vi "labview_program_zfp_interferrometer.vi"() -> ()   [LabVIEW 2015]
uses:
  <vilib>/userdefined/High Color/IMAQdx.ctl
  <vilib>/vision/Image Controls.llb/IMAQ Image.ctl
  <vilib>/Analysis/6fits.llb/Confidence Interval (Linear).vi
  <vilib>/Utility/file.llb/Write Delimited Spreadsheet (DBL).vi
  <vilib>/Analysis/3filter.llb/Butterworth Filter (DBL).vi
  <vilib>/vision/driver/NI_Vision_Acquisition_Software.lvlib
  <resource>/objmgr/imaqdx.rc
  <vilib>/Analysis/NI_AALBase.lvlib
  <vilib>/Analysis/NI_AAL_SigProc.lvlib
  <vilib>/Analysis/NI_AALPro.lvlib
  <vilib>/ptbypt/NI_PtbyPt.lvlib
panel:
  in  "file path (use dialog)":path
  in  "prompt (Choose or enter file path)":string
  out "Intensity Graph":dbl[][](graph)
  in  "y_length":i32=700
  in  "y_axis slicing":i32=30
  in  "x_length":i32=960
  in  "x_axis slicing":i32=10
  out "RawImage":T1(plugin-control)
  in  "Array":dbl[](array[numeric])
  in  "reset graph":bool
  in  "Camera property":bool
  out "gin2":dbl
  in  "sampling freq: fs":dbl=1.0 format="%0.2f"
  out "count":dbl
  out "loop time":u32
  in  "Image Type":T2 items=["Grayscale (U8)", "Grayscale (I16)", "Grayscale (SGL)", "Complex (CSG)", "RGB (U32)", "HSL (U32)", "RGB (U64)", "Grayscale (U16)"]
  out "vert intercept":dbl
  out "vrt. slope":dbl format="%#_9g"
  out "initial array horz":ext[](array[numeric])
  out "initila array horz. fringe":ext[](array[numeric])
  out "Image Out":T1
  in  "?":enum32{"Page 1"}(tab)
  in  "no. of avg":i32=10
  in  "stop":bool
  in  "Session In":T3
  in  "width":i32=4 min=3
  in  "calibration factor vert. fringe":dbl=2000.0
  in  "threshold":dbl=2.0 format="%0.2f"
  in  "sample length":i32=10
  in  "confidence level":dbl=0.95 format="%.2f"
  out "?":string
  out "averaged fringes":dbl[](graph)
  out "Zeroth fringe positon":dbl[](graph)
  in  "image depth (bits)":string(combo)="8 bit"
  in  "contrast":dbl(slide) scale=0.0..5.0 scale format="%#_12g"
  in  "exposure":ext(slide) scale=0.000122070313..0.5 scale format="%#_12g"
  in  "Gain":ext(slide) scale=1.0..200.0
  in  "saturation":u32(slide)=27 scale=0.0..128.0
  in  "order":i32=1
  out "error out":errorcluster
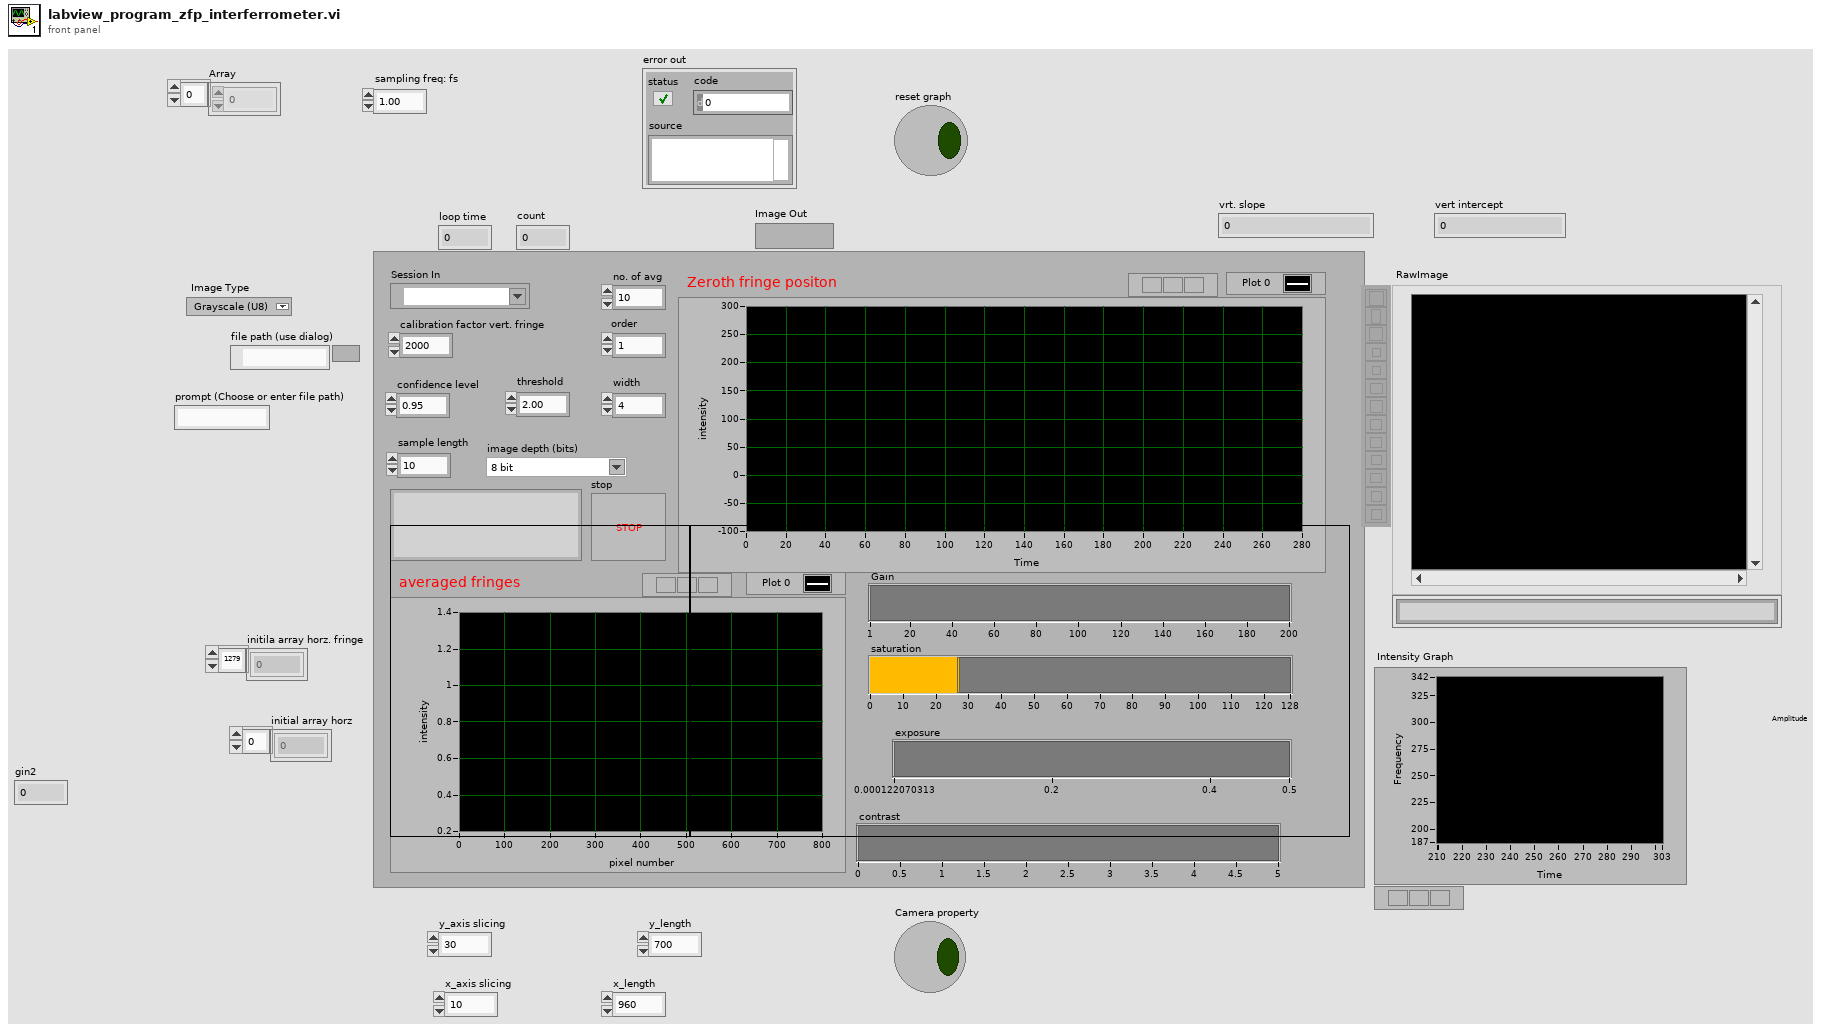
[diagram p1: front panel]
types:
  T1 = typedef "IMAQ Image.ctl" = refnum<image>
  T2 = typedef "Image Type" = u32
  T3 = typedef "IMAQdx.ctl" = refnum<k21>
  T4 = enum16{"open", "replace", "create", "open or create", "replace or create", "replace or create with confirmation"}
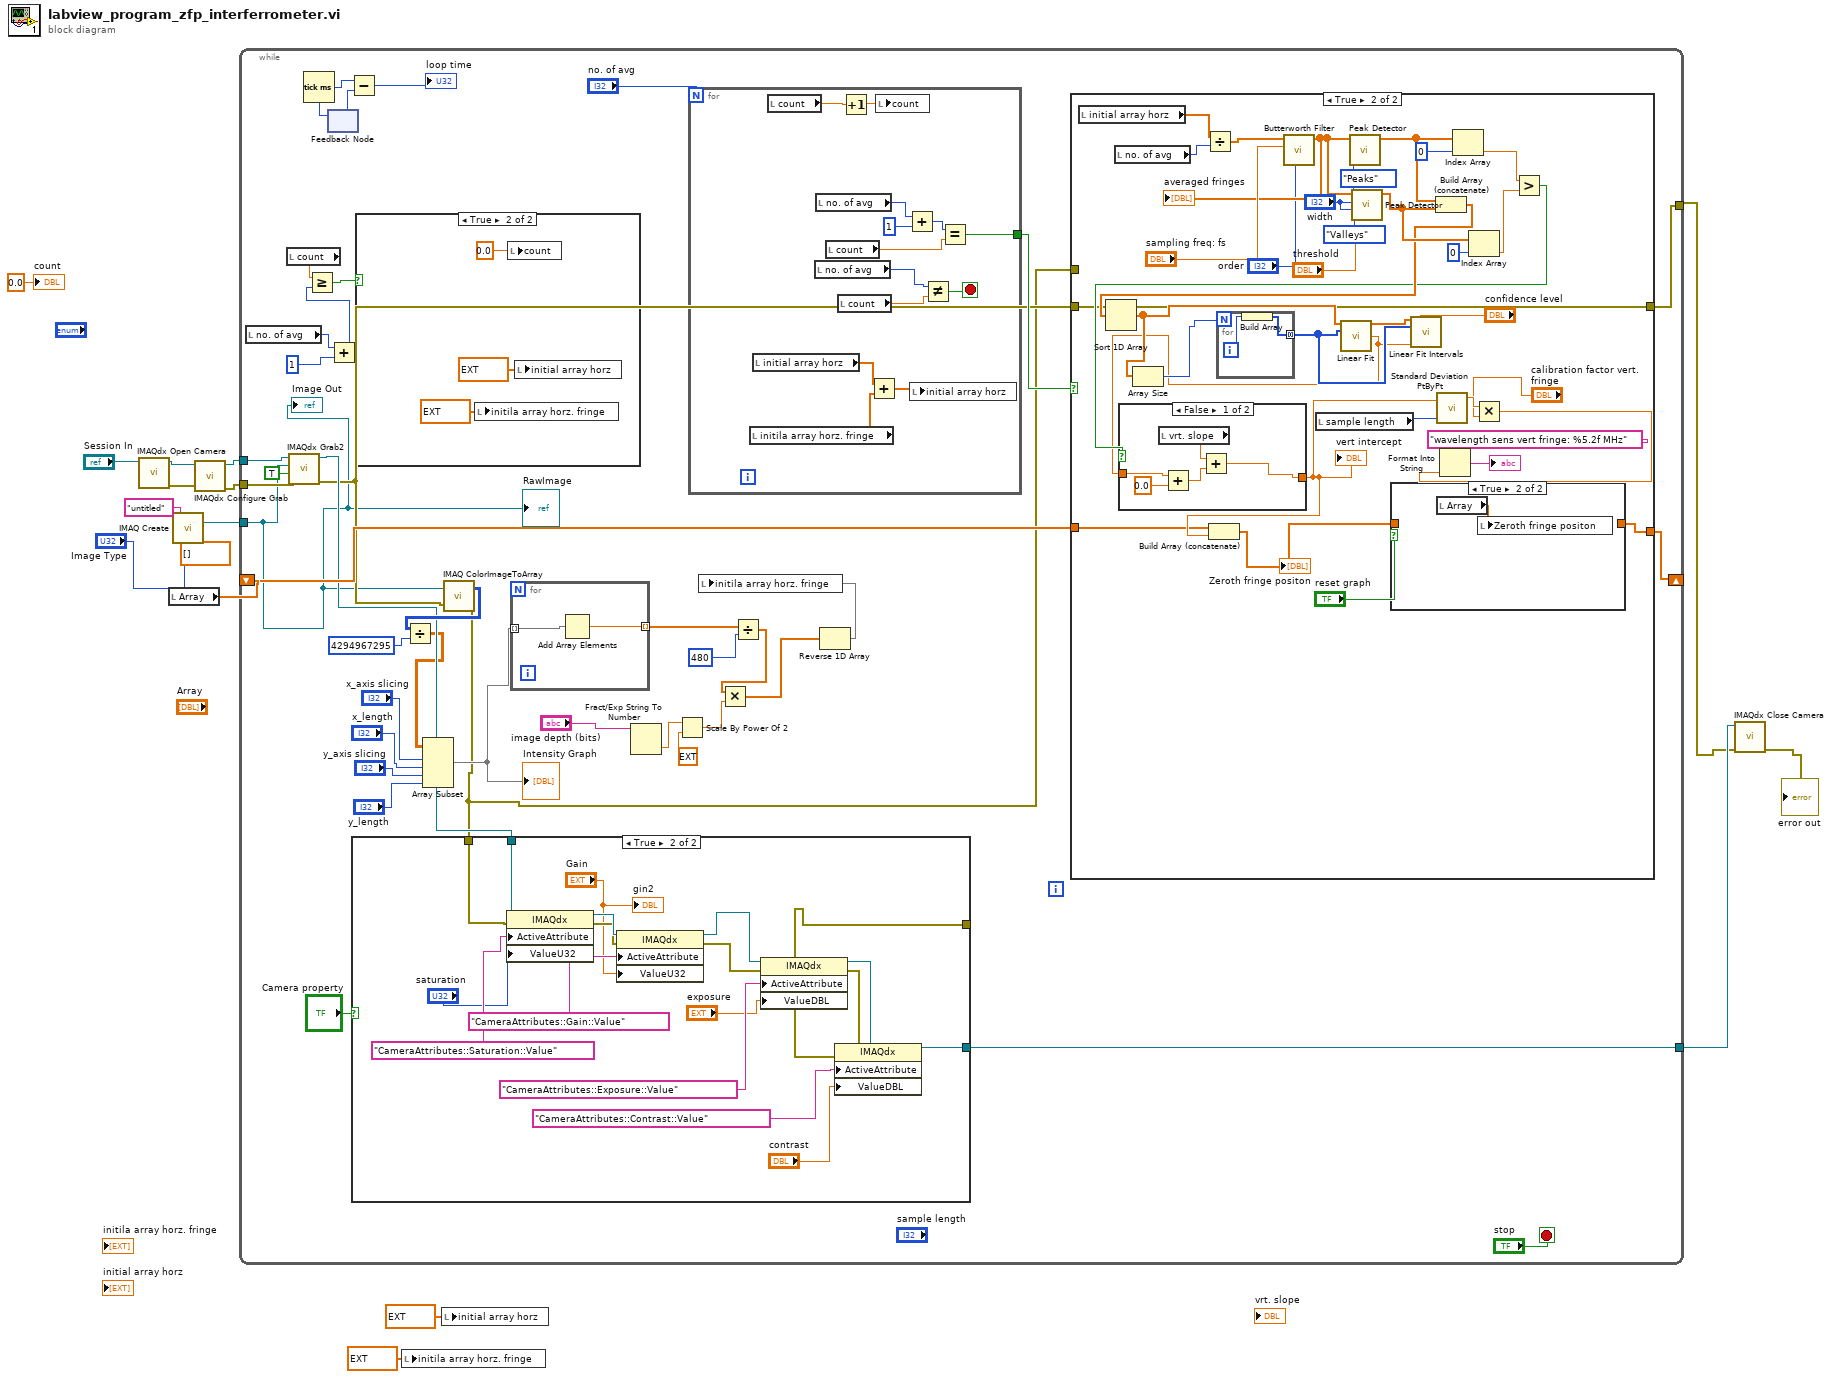
[diagram p0: block diagram]
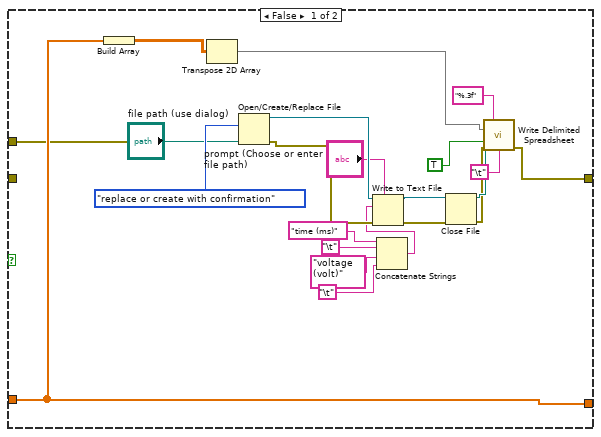
[diagram p4: hidden frame]
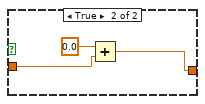
[diagram p6: hidden frame]
diagram:
  (unwired) dbl[] []
  n1 = call <vilib>:"IMAQdx Open Camera.vi"("Session In"="Session In") -> ("error out"=w11:errorcluster, "Session Out"=w12:T3)  [unwired: 9 in]
  n2 = local read "Array"() -> (w4:dbl[])
  n3 = call "IMAQ Create"("Image Name"="untitled", "Image Type"="Image Type") -> ("New Image"=w7:T1)  [unwired: 3 in, 1 out]
  n4 = call <vilib>:"IMAQdx Configure Grab.vi"("error in"=w11, "Session In"=w12) -> ("error out"=w8:errorcluster, "Session Out"=w9:T3)  [unwired: 8 in]
  n5 = while {
    tunnel: [w20] -> w2
    tunnel: w9 -> [w44]
    tunnel: w8 -> [w43]
    tunnel: w7 -> [w16]
    shift-right: [w27] -> _
    shift-left: w4 -> [w39]
    tunnel: [w18] -> w3
    stop <- "stop" stop-if-true
    n6 = local read "no. of avg"() -> (w46:i32)
    n7 = local read "count"() -> (w48:dbl)
    n8 = call <vilib>:"IMAQdx Grab2.vi"("error in"=w43, "Wait for Next Buffer? (Yes)"=TRUE, "Image In"=w16, "Session In"=w44) -> ("error out"=w19:errorcluster, "Session Out"=w36:T3)  [unwired: 4 in, 2 out]
    n9 = Tick Count (ms)() -> (millisecond timer value=w52:u32)
    n10 = feedback #1() -> (w53:u32)  [unwired: 1 in]
    n11 = feedback-in #1(w52) -> ()
    n12 = Add(x=w46, y=1) -> (x+y=w47:i32)
    n13 = Greater Or Equal?(x=w48, y=w47) -> (x >= y?=w49:bool)
    n14 = Subtract(x=w52, y=w53) -> (x-y=→"loop time":u32)
    n15 = case shown="True" w49 {
      frame False {
      }
      frame True {
        n16 = local write "initila array horz. fringe"(ext[] array[1261 elements] ("initila array horz. fringe")) -> ()
        n17 = local write "count"(0.0 ("count")) -> ()
        n18 = local write "initial array horz"(ext[] array[1261 elements] ("initial array horz")) -> ()
      }
    }
    n19 = call "IMAQ ColorImageToArray"("Image"=w16, "error in (no error)"=w19) -> ("Image Pixels (U32)"=w42:u32[][], "error out"=w17:errorcluster)  [unwired: 2 in, 1 out]
    n20 = case shown="True" "Camera property" {
      tunnel: w36 -> [w57 w75]
      tunnel: w17 -> [w56 w72]
      tunnel: [w57 w60] -> w18
      tunnel: [w56 w59] -> _
      frame False {
      }
      frame True {
        n21 = property class="IMAQdx"(reference=w75, error in=w72, "ActiveAttribute"="CameraAttributes::Saturation::Value", "ValueU32"="saturation") -> (reference out=w71:T3, error out=w70:errorcluster)
        n22 = property class="IMAQdx"(reference=w71, error in=w70, "ActiveAttribute"="CameraAttributes::Gain::Value", "ValueU32"="Gain") -> (reference out=w66:T3, error out=w67:errorcluster)
        n23 = property class="IMAQdx"(reference=w66, error in=w67, "ActiveAttribute"="CameraAttributes::Exposure::Value", "ValueDBL"="exposure") -> (reference out=w63:T3, error out=w62:errorcluster)
        n24 = property class="IMAQdx"(reference=w63, error in=w62, "ActiveAttribute"="CameraAttributes::Contrast::Value", "ValueDBL"="contrast") -> (reference out=w60:T3, error out=w59:errorcluster)
        "gin2" <- "Gain"
      }
    }
    n25 = Divide(x=w42, y=u32 4294967295) -> (x/y=w22:dbl[][])
    n26 = Array Subset(array=w22, index (row)="x_axis slicing", length (row)="x_length", index (col)="y_axis slicing", length (col)="y_length") -> (w21:dbl[][])
    "Intensity Graph" <- w21
    n27 = for {
      tunnel: w21 -> [w77] mode=indexing
      tunnel: [w76] -> w40 mode=indexing
      n28 = Add Array Elements(numeric array=w77) -> (sum=w76:dbl)
    }
    n29 = Fract/Exp String To Number(string="image depth (bits)") -> (number=w32:dbl)  [unwired: 3 in, 1 out]
    n30 = Scale By Power Of 2(n=w32, x=ext 1.0) -> (x*2^n=w31:ext)
    n31 = for {
      N: "no. of avg" -> [_]
      tunnel: [w157] -> w50
      stop <- w161 stop-if-true
      n32 = local read "initila array horz. fringe"() -> (w151:ext[])
      n33 = local read "initial array horz"() -> (w153:ext[])
      n34 = local read "count"() -> (w163:dbl)
      n35 = local read "no. of avg"() -> (w160:i32)
      n36 = local read "no. of avg"() -> (w156:i32)
      n37 = local read "count"() -> (w158:dbl)
      n38 = local read "count"() -> (w159:dbl)
      n39 = Increment(x=w163) -> (x+1=w162:dbl)
      n40 = Add(x=w153, y=w151) -> (x+y=w152:ext[])
      n41 = local write "count"(w162) -> ()
      n42 = Add(x=w156, y=1) -> (x+y=w154:i32)
      n43 = local write "initial array horz"(w152) -> ()
      n44 = Not Equal?(x=w160, y=w159) -> (x != y?=w161:bool)
      n45 = Equal?(x=w154, y=w158) -> (x = y?=w157:bool)
    }
    n46 = Divide(x=w40, y=480) -> (x/y=w29:dbl[])
    n47 = Multiply(x=w29, y=w31) -> (x*y=w28:ext[])
    n48 = Reverse 1D Array(array=w28) -> (reversed array=w37:ext[])
    n49 = local write "initila array horz. fringe"(w37) -> ()
    n50 = case shown="True" w50 {
      tunnel: [w84 w105] -> w27
      tunnel: w39 -> [w84 w111]
      tunnel: [w82 w103] -> w20
      tunnel: w19 -> [_ w103]
      tunnel: w17 -> [w81 _]
      frame False {
        n51 = Build Array(w84) -> (w83:dbl[][])
        n52 = Transpose 2D Array(2D array=w83) -> (transposed array=w99:dbl[][])
        n53 = Open/Create/Replace File(file path (use dialog)="file path (use dialog)", error in=w81, operation (0:open)=T4."replace or create with confirmation") -> (refnum out=w102:refnum<file>, error out=w101:errorcluster)  [unwired: 3 in, 1 out]
        n54 = Concatenate Strings("time (ms)" ("string"), "\t", "voltage (volt)" ("string"), "\t") -> (w94:string)
        n55 = Write to Text File(prompt (Choose or enter file path)="prompt (Choose or enter file path)", file (use dialog)=w102, text=w94, error in=w101) -> (refnum out=w96:refnum<file>, error out=w95:errorcluster)  [unwired: 1 out]
        n56 = Close File(refnum=w96, error in=w95) -> (path=w90:path, error out=w87:errorcluster)
        n57 = call-poly <vilib>:"Write Delimited Spreadsheet.vi"("file path (dialog if empty)"=w90, "format (%.3f)"="%.3f", "2D data"=w99, "append to file? (F)"=TRUE ("append to file? (new file:F)"), "error in (no error)"=w87, "delimiter (\\t)"="\t") -> ("error out"=w82:errorcluster)  [unwired: 8 in, 1 out]
      }
      frame True {
        n58 = local read "initial array horz"() -> (w138:ext[])
        n59 = local read "no. of avg"() -> (w137:i32)
        n60 = Divide(x=w138, y=w137) -> (x/y=w136:ext[])
        n61 = call-poly <vilib>:"Butterworth Filter.vi"("order"="order", "sampling freq: fs"="sampling freq: fs", "X"=w136) -> ("Filtered X"=w108:dbl[])  [unwired: 5 in, 1 out]
        "averaged fringes" <- w108
        n62 = local read "sample length"() -> (w117:i32)
        n63 = call <vilib>:"Peak Detector.vi"("peaks/valleys"=enum32{"Peaks", "Valleys"}."Peaks", "width"="width", "X"=w108) -> ("Locations"=w130:dbl[])  [unwired: 4 in, 4 out]
        n64 = call <vilib>:"Peak Detector.vi"("peaks/valleys"=enum32{"Peaks", "Valleys"}."Valleys", "width"="width", "threshold"="threshold", "X"=w108) -> ("Locations"=w131:dbl[])  [unwired: 3 in, 4 out]
        n65 = Build Array (concatenate)(w130, w131) -> (w125:dbl[])
        n66 = Sort 1D Array(array=w125) -> (sorted array=w123:dbl[])
        n67 = Array Size(array=w123) -> (size(s)=w124:i32)
        n68 = for {
          N: w124 -> [_]
          tunnel: [w150] -> w120 mode=concatenating
          i -> [w149]
          n69 = Build Array(w149) -> (w150:i32[])
        }
        n70 = call <vilib>:"Linear Fit.vi"("Y"=w123, "X"=w120) -> ("Best Linear Fit"=w121:dbl[], "intercept"=w119:dbl)  [unwired: 9 in, 3 out]
        n71 = call-poly <vilib>:"Linear Fit Intervals.vi"("Y"=w121, "confidence level"="confidence level", "X"=w120, "intercept"=w119) -> ()  [unwired: 7 in, 5 out]
        n72 = Index Array(array=w130, index=0) -> (element=w127:dbl)
        n73 = Index Array(array=w131, index=0) -> (element=w126:dbl)
        n74 = Greater?(x=w127, y=w126) -> (0:w122:bool)
        n75 = case shown="False" w122 {
          tunnel: [w145 w148] -> w112
          tunnel: w119 -> [w141 w146]
          frame False {
            n76 = local read "vrt. slope"() -> (w144:dbl)
            n77 = Add(x=w141, y=0.0) -> (x+y=w143:dbl)
            n78 = Add(x=w144, y=w143) -> (x+y=w145:dbl)
          }
          frame True {
            n79 = Add(x=0.0, y=w146) -> (x+y=w148:dbl)
          }
        }
        "vert intercept" <- w112
        n80 = Build Array (concatenate)(w111, w112) -> (w104:dbl[])
        "Zeroth fringe positon" <- w104
        n81 = case shown="True" "reset graph" {
          tunnel: [w139 _] -> w105
          tunnel: w104 -> [w139 _]
          frame False {
          }
          frame True {
            n82 = local read "Array"() -> (w140:dbl[])
            n83 = local write "Zeroth fringe positon"(w140) -> ()
          }
        }
        n84 = call <vilib>:"Standard Deviation PtByPt.vi"("x"=w112, "sample length"=w117) -> ("standard deviation"=w116:dbl)  [unwired: 1 in, 2 out]
        n85 = Multiply(x=w116, y="calibration factor vert. fringe") -> (x*y=w110:dbl)
        n86 = Format Into String(format string="wavelength sens vert fringe: %5.2f MHz", w110) -> (resulting string=→"?":string)  [unwired: 2 in, 1 out]
      }
    }
    "Image Out" <- w16
    "RawImage" <- w16
  }
  n87 = local write "initila array horz. fringe"(ext[] array[1261 elements] ("initila array horz. fringe")) -> ()
  n88 = local write "initial array horz"(ext[] array[1261 elements] ("initial array horz")) -> ()
  n89 = call <vilib>:"IMAQdx Close Camera.vi"("error in"=w2, "Session In"=w3) -> ("error out"=→"error out":errorcluster)  [unwired: 9 in]
  "count" <- 0.0 ("count")
